vi "FetchIncrementFile.vi"(10 "extension":string="tif", 11 "name":string="myname") -> (1 "path":path)   [LabVIEW 2018, in "RW_Protocols.lvlib"]
uses:
  RW_Protocols.lvlib
  DefaultSavingPath.vi
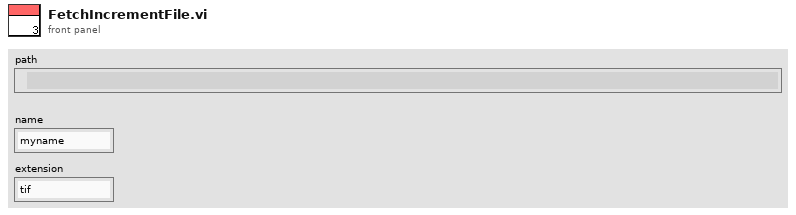
[diagram p1: front panel]
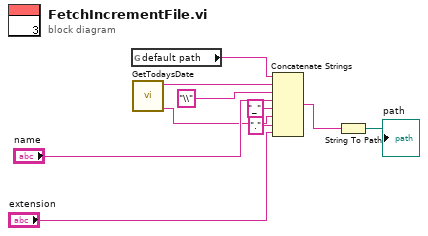
[diagram p0: block diagram]
diagram:
  n1 = global read "DefaultSavingPath.vi" "default path"() -> (w10:string)
  n2 = call "GetTodaysDate.vi"() -> ("time string"=w6:string, "concatenated string"=w9:string)  [unwired: 10 in]
  n3 = Concatenate Strings(w10, w9, "\\" ("string"), "name", "_" ("string"), w6, "." ("string"), "extension") -> (w2:string)
  n4 = String To Path(string=w2) -> (path=→"path":path)
